vi "ke37xx Timer.vi"(0 "VISA Resource Name":refnum<visa-resource-name>, 7 "Action (0: Measure)":enum16{"Measure", "Reset"}(ring), 11 "error in (no error)":errorcluster) -> (4 "VISA Resource Name Out":refnum<visa-resource-name>, 15 "error out":errorcluster)   [LabVIEW 2009, in "Keithley 3700 Series.lvlib"]
doc: "This VI allows you to use the system timer to measure the time between events. The VI also allows you to reset the timer.\n\nThe value returned represents the elapsed time in seconds since the timer was reset.\nThe returned resolution for time depends on how long it has been since the timer was reset. It starts with 1s resolution and starts to lose resolution after about 2.8 minutes."
uses:
  <instrlib>/Keithley 3706/Keithley 3700 Series.lvlib
panel:
  out "Timer Value":dbl
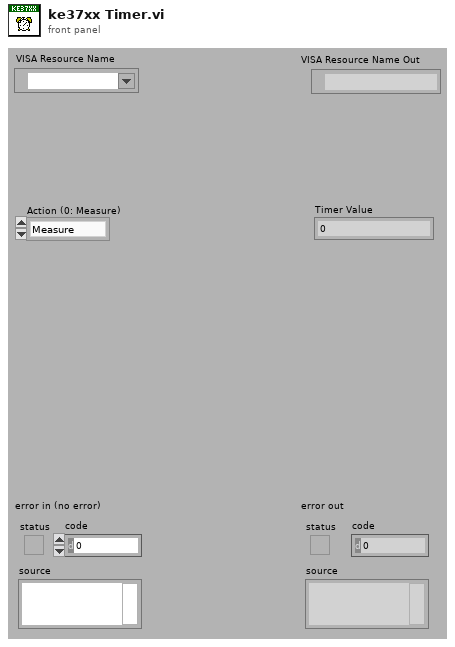
[diagram p1: front panel]
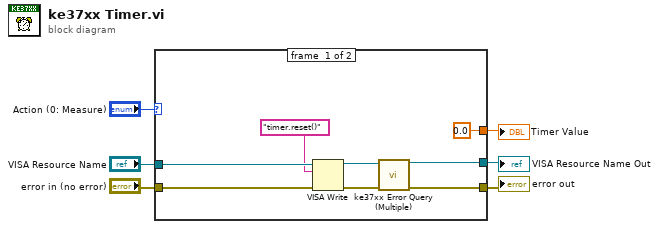
[diagram p0: block diagram]
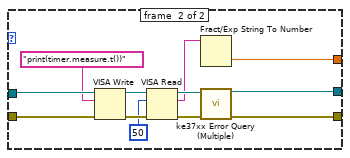
[diagram p2: hidden frame]
diagram:
  n1 = case shown="\"Measure\"" "Action (0: Measure)" {
    tunnel: "VISA Resource Name" -> [w14 w26]
    tunnel: "error in (no error)" -> [w13 w25]
    tunnel: [w12 w24] -> w4
    tunnel: [w11 w23] -> w3
    tunnel: [0.0 w15] -> w1
    frame #0 {
      n2 = VISA Write(VISA resource name=w14, write buffer="timer.reset()", error in (no error)=w13) -> (VISA resource name out=w10:refnum<visa-resource-name>, error out=w9:errorcluster)  [unwired: 1 out]
      n3 = call <instrlib>:"ke37xx Error Query (Multiple).vi"("VISA resource name"=w10, "error in (no error)"=w9) -> ("VISA resource name out"=w12:refnum<visa-resource-name>, "error out"=w11:errorcluster)  [unwired: 12 out]
    }
    frame #1 {
      n4 = VISA Write(VISA resource name=w26, write buffer="print(timer.measure.t())", error in (no error)=w25) -> (VISA resource name out=w21:refnum<visa-resource-name>, error out=w22:errorcluster)  [unwired: 1 out]
      n5 = VISA Read(VISA resource name=w21, byte count=u32 50, error in (no error)=w22) -> (VISA resource name out=w20:refnum<visa-resource-name>, read buffer=w17:string, error out=w19:errorcluster)  [unwired: 1 out]
      n6 = Fract/Exp String To Number(string=w17) -> (number=w15:dbl)  [unwired: 4 out]
      n7 = call <instrlib>:"ke37xx Error Query (Multiple).vi"("VISA resource name"=w20, "error in (no error)"=w19) -> ("VISA resource name out"=w24:refnum<visa-resource-name>, "error out"=w23:errorcluster)  [unwired: 12 out]
    }
  }
  "VISA Resource Name Out" <- w4
  "error out" <- w3
  "Timer Value" <- w1
